vi "test Add-Get Bus Status Section.vi"(8 "error in":errorcluster, 11 "TestCase in":refnum<class "Scripting.lvclass">) -> (0 "error out":errorcluster, 3 "TestCase out":refnum<class "Scripting.lvclass">)   [LabVIEW 2020, in "Scripting.lvclass"]
uses:
  Scripting.lvclass
  <vilib>/addons/_JKI Toolkits/VI Tester/TestCase.llb/TestCase.lvclass
  Scripting/AIM MIL-STD-1553 Scripting.lvlib
  C:/dev/git/niveristand-custom-device-testing-tools/VeriStandScriptingTestCase/VeriStandScriptingTestCase.lvclass
  C:/Program Files (x86)/National Instruments/LabVIEW 2020/vi.lib/addons/_JKI Toolkits/VI Tester/TestCase.llb/TestCase.lvclass
  C:/dev/git/niveristand-aim-milStd1553-custom-device/Source/Custom Device Support/Tests/Unit/Scripting/Scripting.lvclass
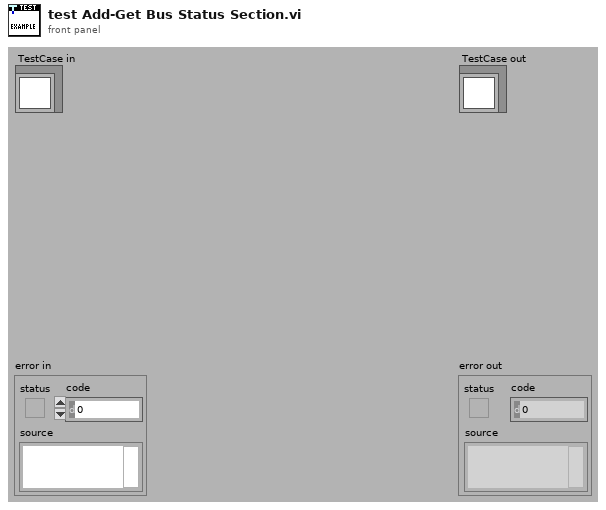
[diagram p1: front panel]
types:
  T1 = typedef "Custom Device API.lvlib/Custom Device Item Ref.ctl" = u64
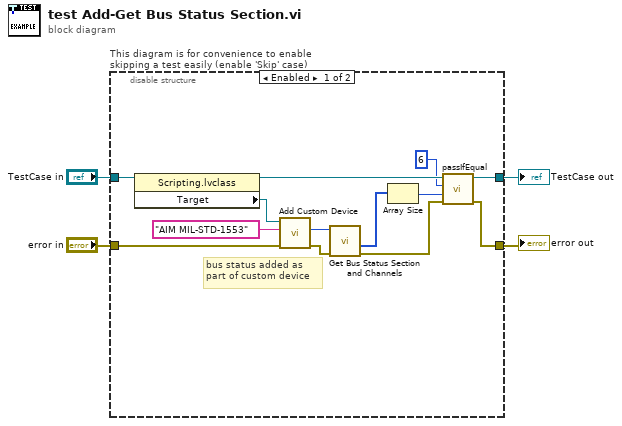
[diagram p0: block diagram]
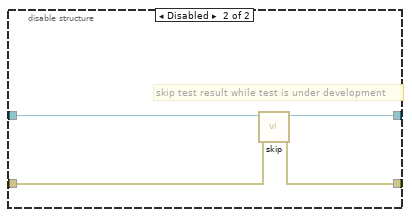
[diagram p2: hidden frame]
diagram:
  n1 = disable-structure "This diagram is for convenience to enable skipping a test easily (enable 'Skip' case)" shown="Enabled" {
    disable-tunnel: "TestCase in" -> [w15 w21]
    disable-tunnel: [w12 w19] -> w1
    disable-tunnel: [w5 w20] -> w3
    disable-tunnel: "error in" -> [w17 w18]
    frame Enabled {
      # "bus status added as part of custom device"
      n2 = property class="Scripting.lvclass"(reference=w15) -> (reference out=w13:refnum<class "Scripting.lvclass">, "Target"=w14:refnum<k24>)  [unwired: 1 in, 1 out]
      n3 = call "Add Custom Device.vi"("error in"=w17, "custom device name"="AIM MIL-STD-1553" ("name"), "target"=w14) -> ("error out"=w11:errorcluster, "custom device"=w10:T1)  [unwired: 6 in, 1 out]
      n4 = call "Get Bus Status Section and Channels.vi"("error in"=w11, "custom device"=w10) -> ("error out"=w8:errorcluster, "bus status channels"=w9:T1[])  [unwired: 5 in, 3 out]
      n5 = Array Size(array=w9) -> (size(s)=w7:i32)
      n6 = call-dynamic "passIfEqual.vi"("error in (no error)"=w8, "y"=w7, "x"=6 ("size(s)"), "TestCase in"=w13) -> ("error out"=w5:errorcluster, "TestCase out"=w12:refnum<class "Scripting.lvclass">)  [unwired: 6 in]
    }
    frame Disabled {
      # "skip test result while test is under development"
      n7 = call <vilib>:"skip.vi"("error in (no error)"=w18, "TestCase in"=w21) -> ("error out"=w20:errorcluster, "TestCase out"=w19:refnum<class "Scripting.lvclass">)  [unwired: 8 in]
    }
  }
  "error out" <- w3
  "TestCase out" <- w1
